vi "Filter and Data Scaling backup (062609) temp.vi"(0 "Offset Data":string[](array[string]), 1 "FM1 Frequency":dbl format="%#_13g", 5 "Slope Data":string[](array[string]), 7 "Filter Data":string[](array[string]), 9 "Vin":dbl[](array[numeric]), 11 "error in":errorcluster, 12 "Allow Zero?":string[](array[string])) -> (4 "Vout":string[](array[string]), 6 "Offset Data":string[](array[string]), 8 "ScaledOut":string[](array[string]), 10 "ScaledOut":dbl[](array[numeric]), 14 "Allow Zero?":string[](array[string]), 15 "error out":errorcluster)   [LabVIEW 2018]
uses:
  <vilib>/ptbypt/NI_PtbyPt.lvlib
panel:
  # "32-51= FM1 GPM Data Point 1-20"
  # "32-51= FM1 Data Point # 1-20"
  # "32-51 = FM1 K Factor 1-20"
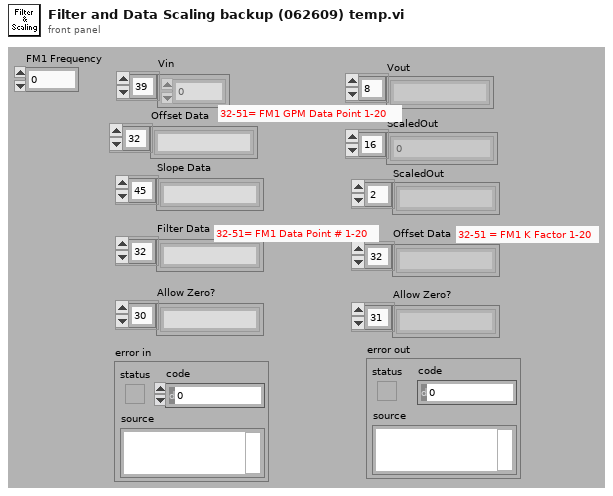
[diagram p1: front panel]
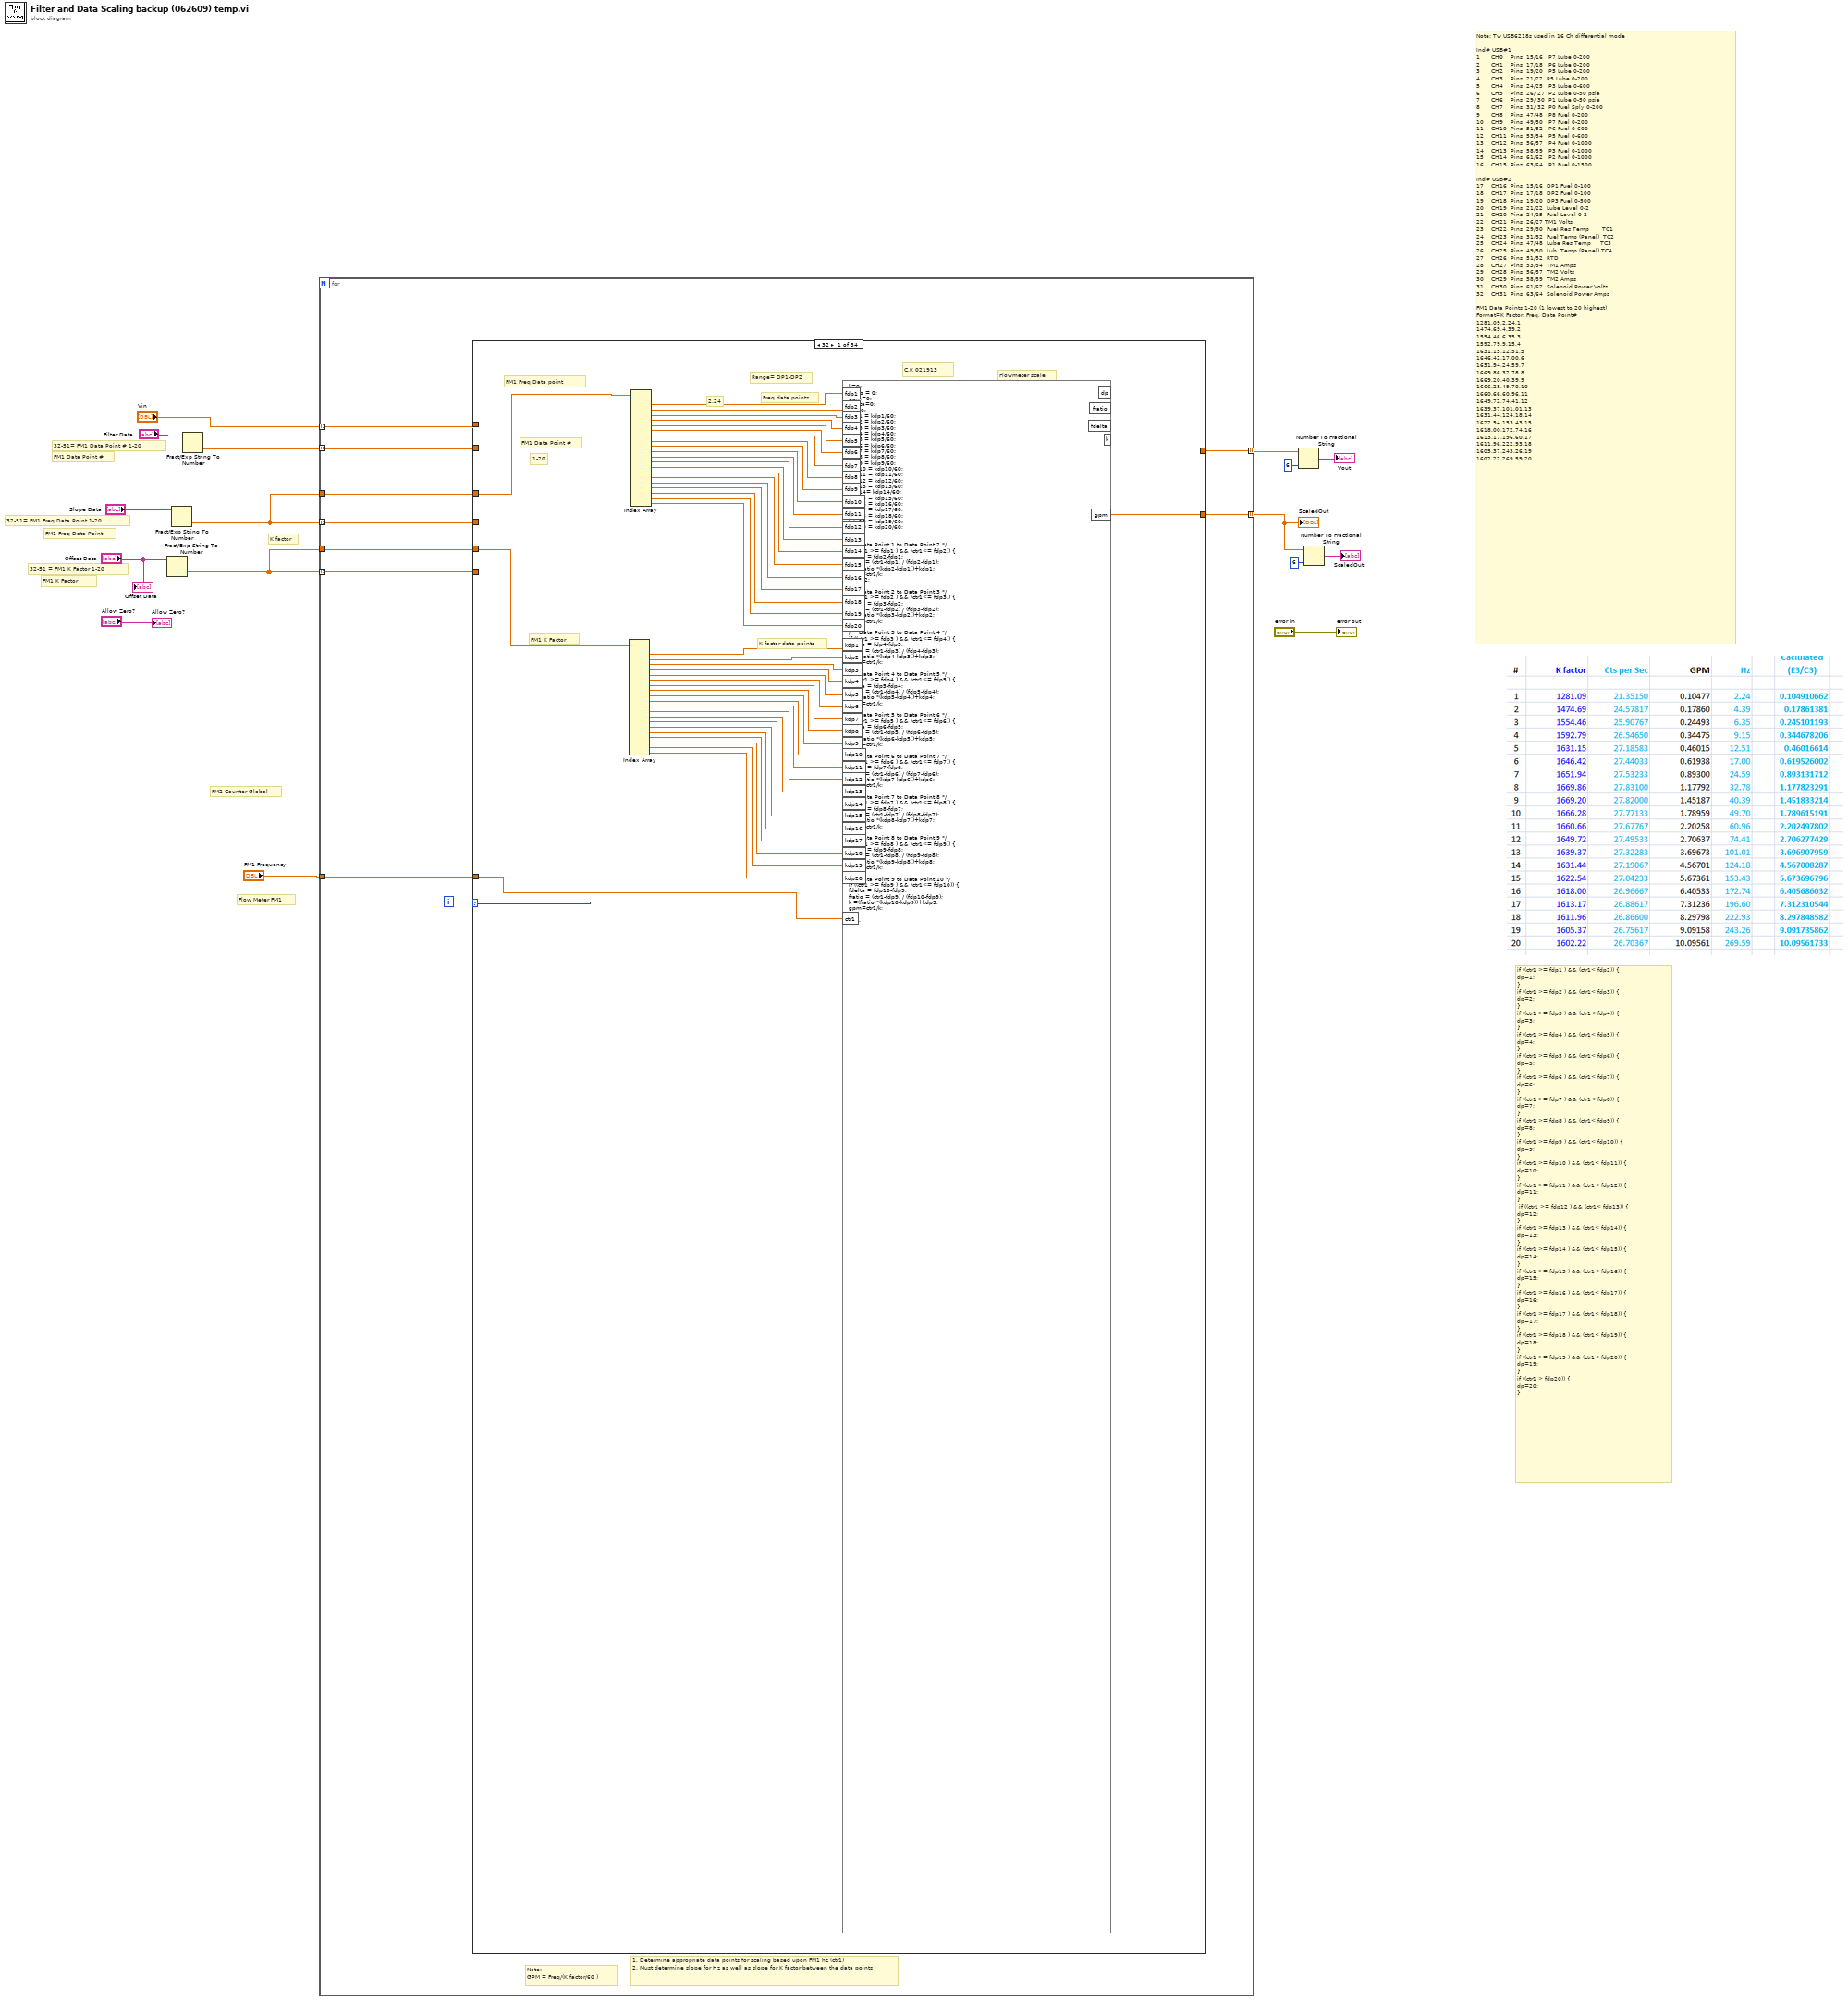
[diagram p0: block diagram]
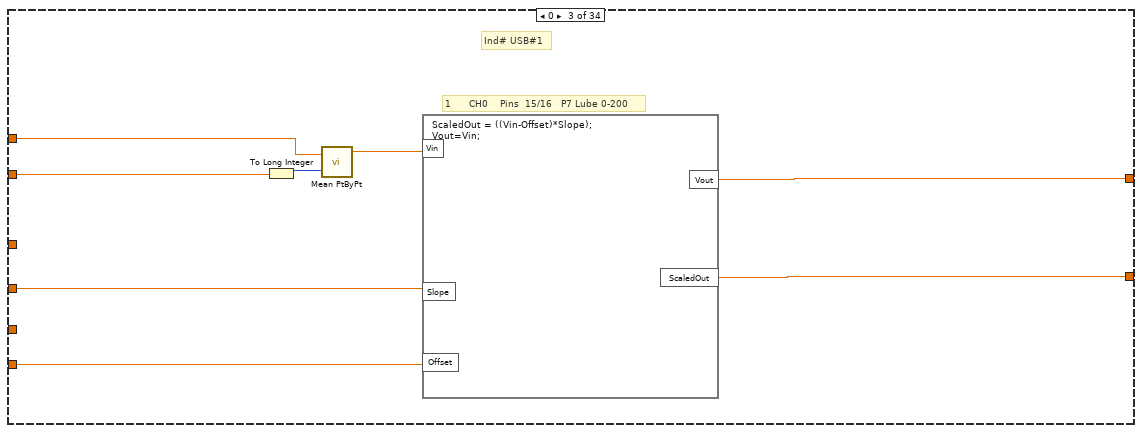
[diagram p3: hidden frame]
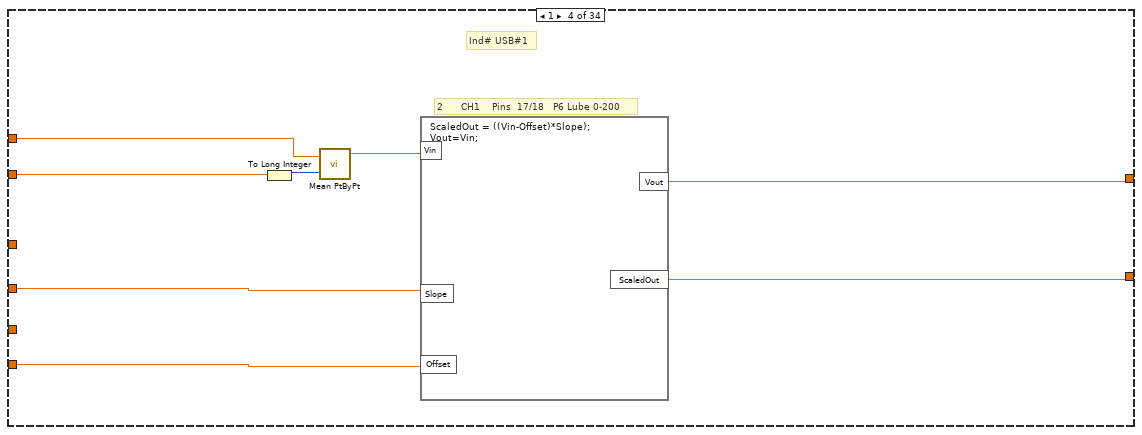
[diagram p4: hidden frame]
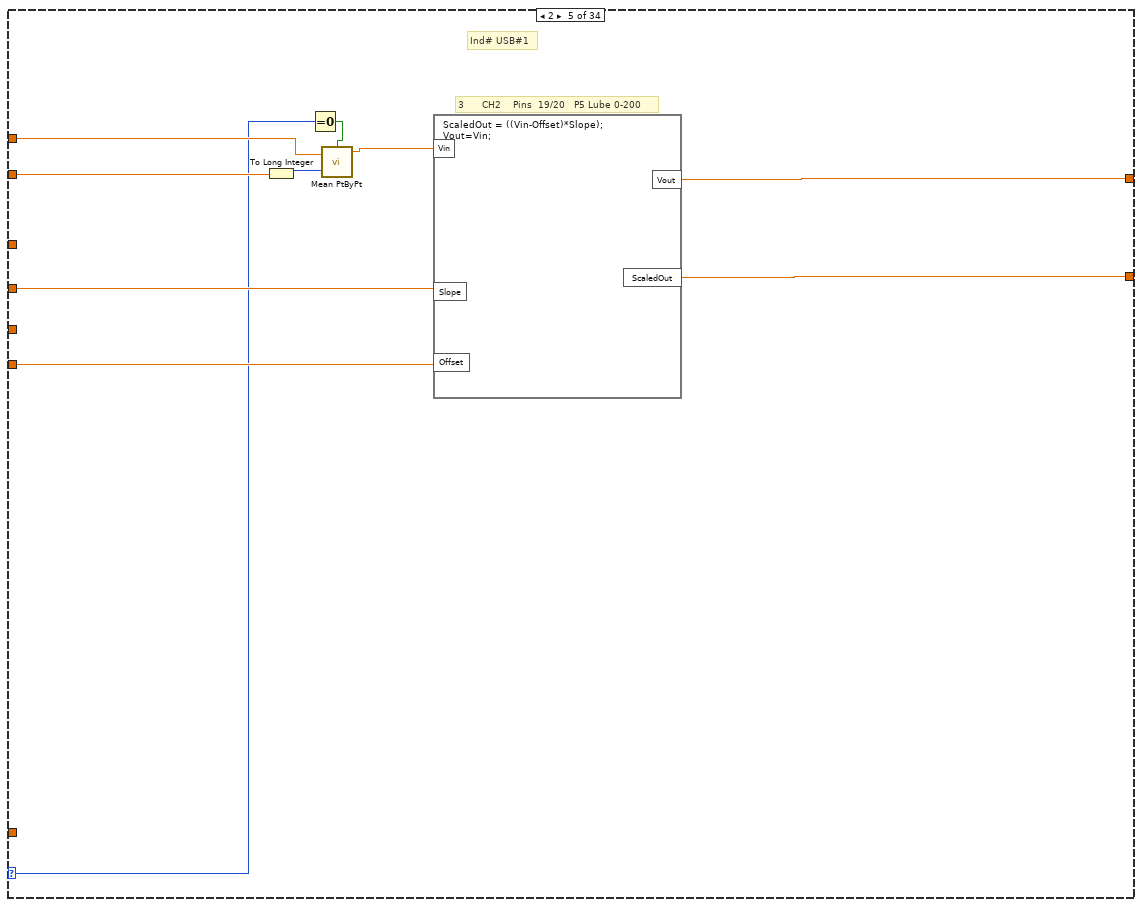
[diagram p5: hidden frame]
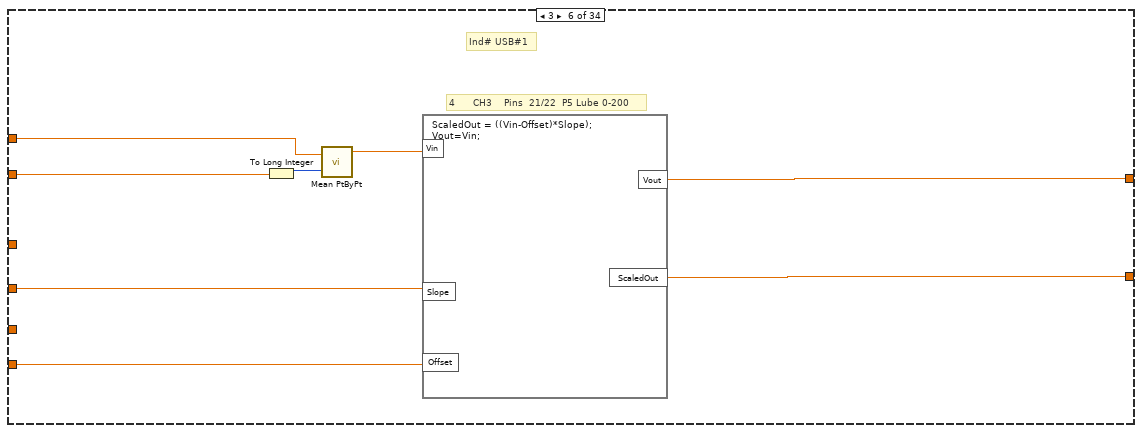
[diagram p6: hidden frame]
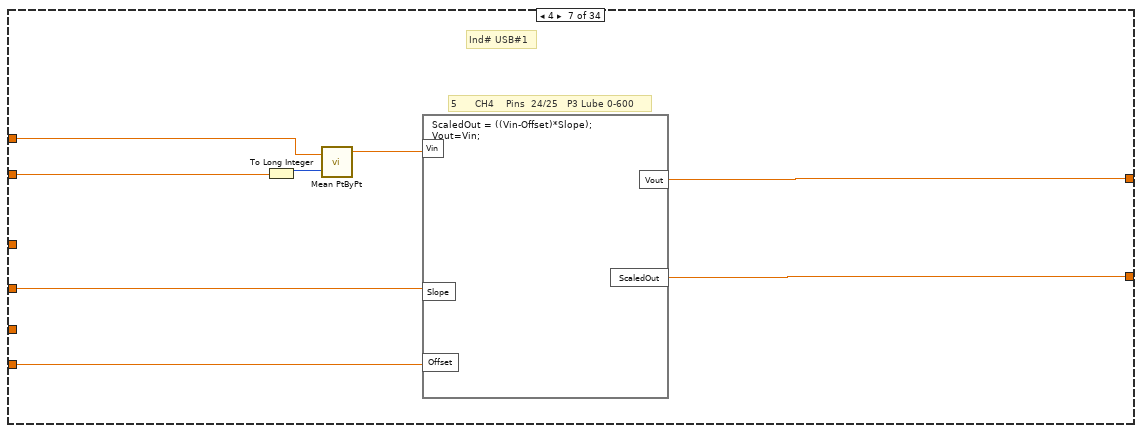
[diagram p7: hidden frame]
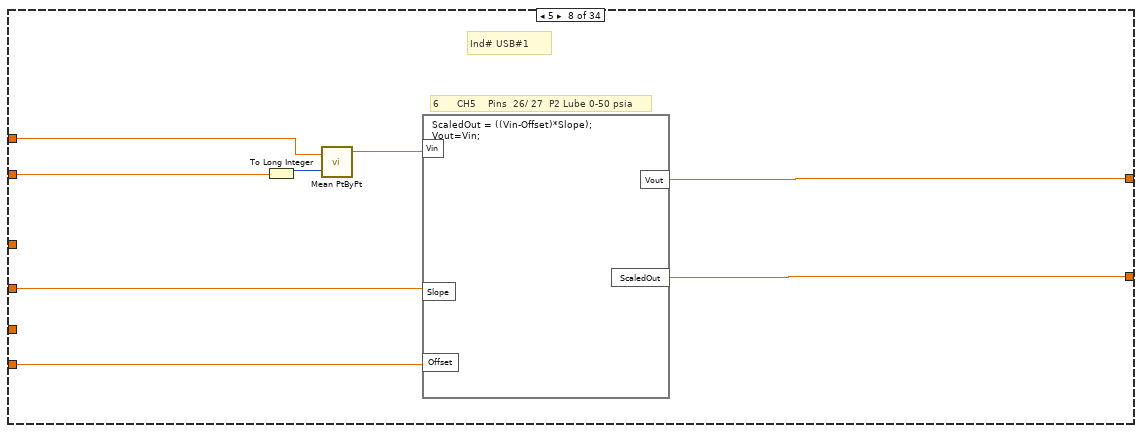
[diagram p8: hidden frame]
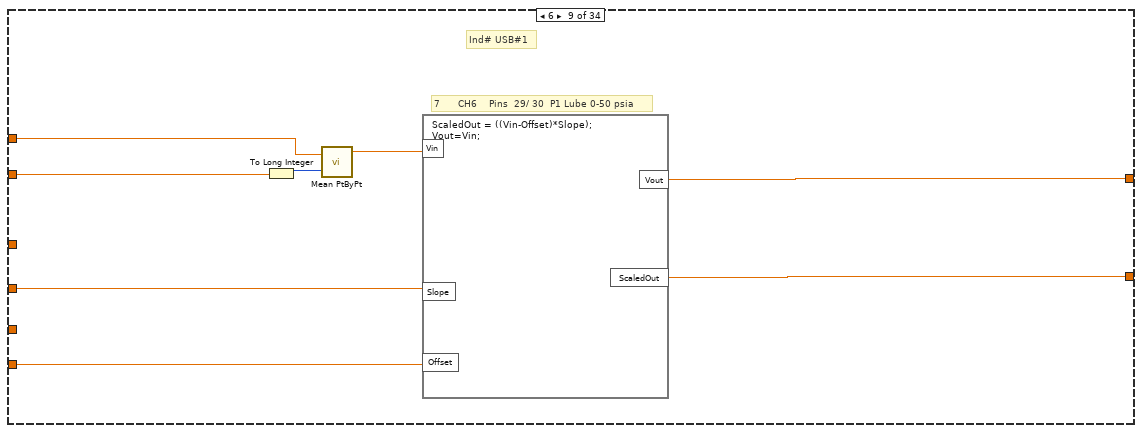
[diagram p9: hidden frame]
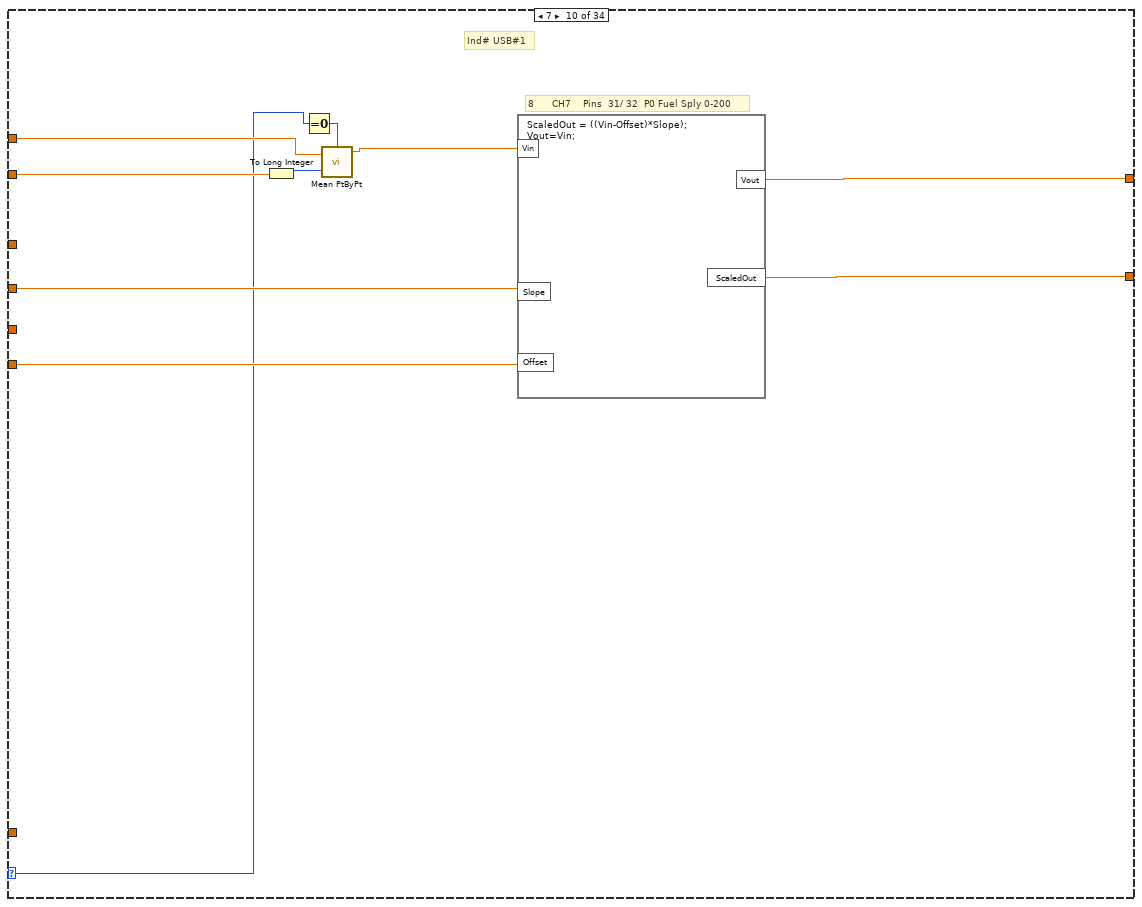
[diagram p10: hidden frame]
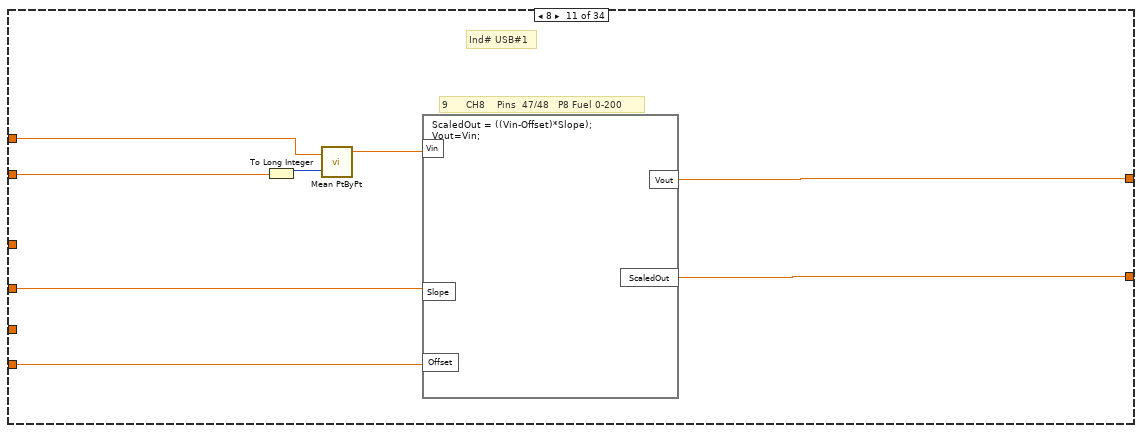
[diagram p11: hidden frame]
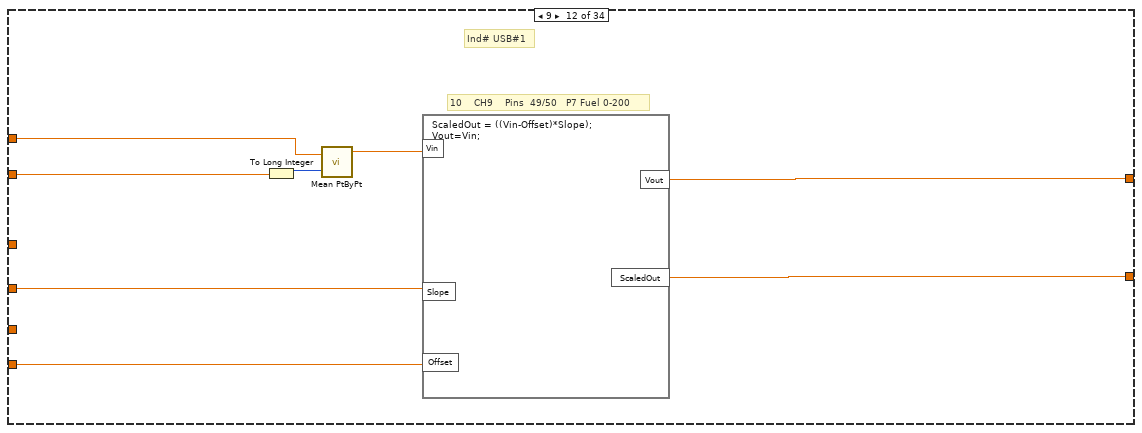
[diagram p12: hidden frame]
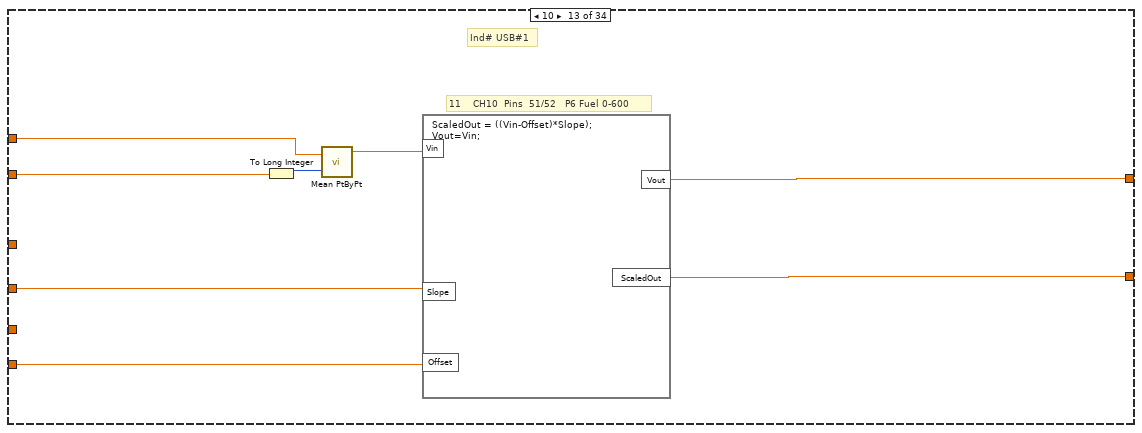
[diagram p13: hidden frame]
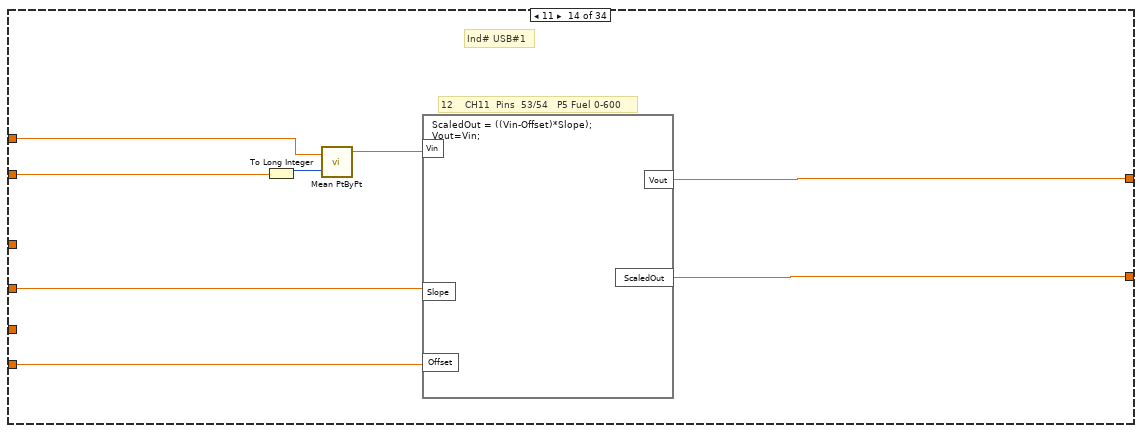
[diagram p14: hidden frame]
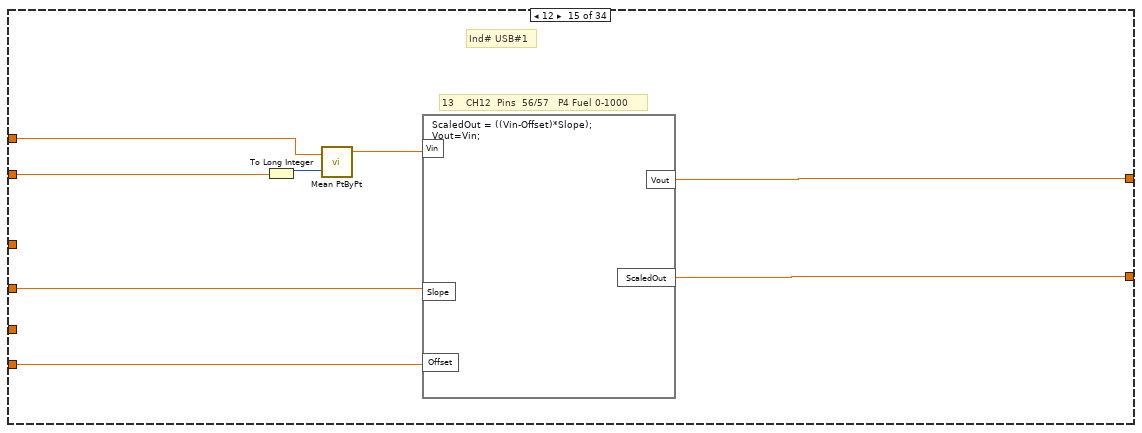
[diagram p15: hidden frame]
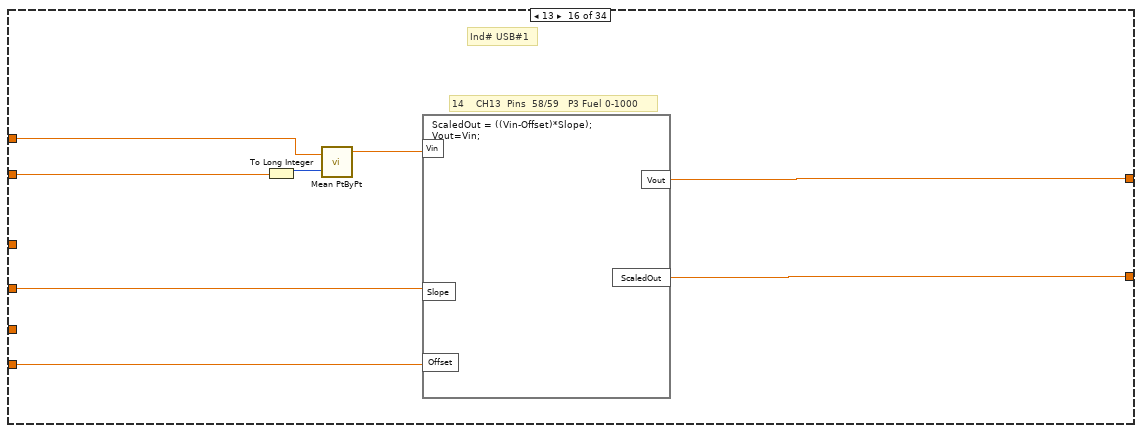
[diagram p16: hidden frame]
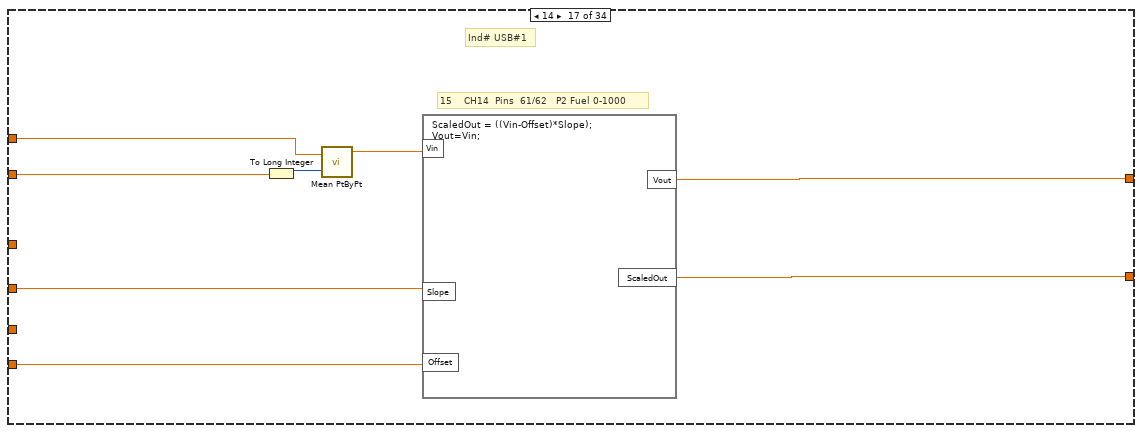
[diagram p17: hidden frame]
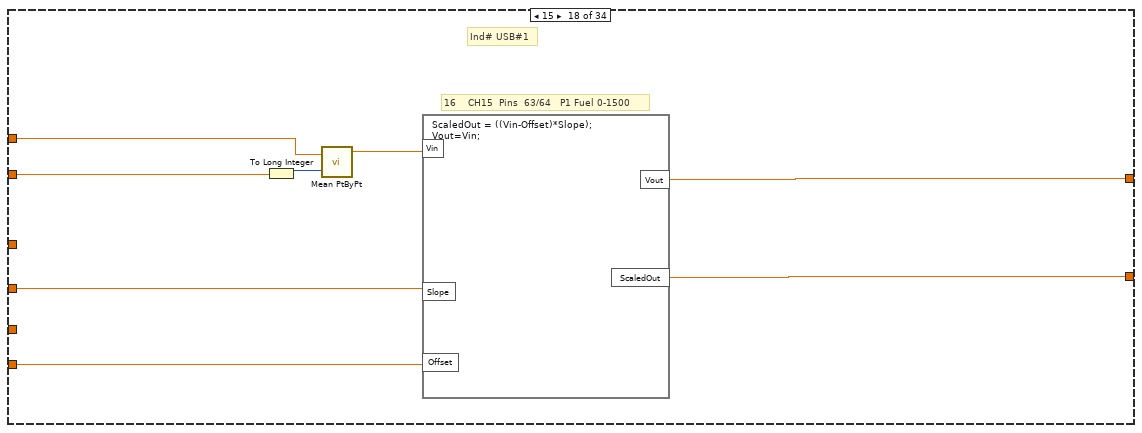
[diagram p18: hidden frame]
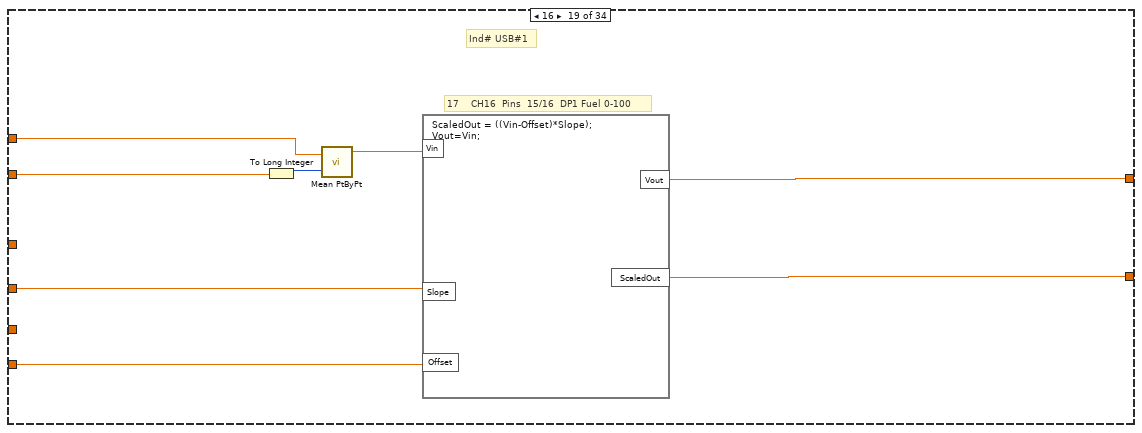
[diagram p19: hidden frame]
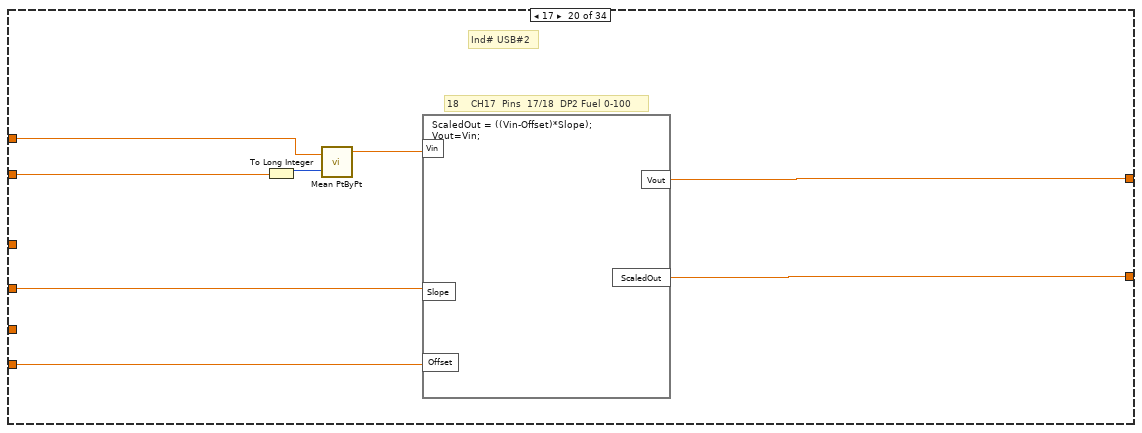
[diagram p20: hidden frame]
diagram:
  # "Flow Meter FM1"
  # "if ((ctr1 >= fdp1 ) && (ctr1< fdp2)) {\ndp=1;\n}\nif ((ctr1 >= fdp2 ) && (ctr1< fdp3)) {\ndp=2;\n}\nif ((ctr1 >= fdp3 ) && (ctr1< fdp4)) {\ndp=3;\n}\nif ((ctr1 >= fdp4 ) && (ctr1< fdp5)) {\ndp=4;\n}\nif ((ctr1 >= fdp5 ) && (ctr1< fdp6)) {\ndp=5;\n}\nif ((ctr1 >= fdp6 ) && (ctr1< fdp7)) {\ndp=6;\n}\nif ((ctr1 >= fdp7 ) && (ctr1< fdp8)) {\ndp=7;\n}\nif ((ctr1 >= fdp8 ) && (ctr1< fdp9)) {\ndp=8;\n}\nif ((ctr1 >= fdp9 ) && (ctr1< fdp10)) {\ndp=9;\n}\nif ((ctr1 >= fdp10 ) && (ctr1< fdp11)) {\ndp=10;\n}\nif ((ctr1 >= fdp11 ) && (ctr1< fdp12)) {\ndp=11;\n}\n if ((ctr1 >= fdp12 ) && (ctr1< fdp13)) {\ndp=12;\n}\nif ((ctr1 >= fdp13 ) && (ctr1< fdp14)) {\ndp=13;\n}\nif ((ctr1 >= fdp14 ) && (ctr1< fdp15)) {\ndp=14;\n}\nif ((ctr1 >= fdp15 ) && (ctr1< fdp16)) {\ndp=15;\n}\nif ((ctr1 >= fdp16 ) && (ctr1< fdp17)) {\ndp=16;\n}\nif ((ctr1 >= fdp17 ) && (ctr1< fdp18)) {\ndp=17;\n}\nif ((ctr1 >= fdp18 ) && (ctr1< fdp19)) {\ndp=18;\n}\nif ((ctr1 >= fdp19 ) && (ctr1< fdp20)) {\ndp=19;\n}\nif ((ctr1 > fdp20)) {\ndp=20;\n}"
  # "Note: Tw USB6218s used in 16 Ch differential mode\n\nInd# USB#1\n1      CH0\t\t  Pins  15/16\t  P7 Lube 0-200\n2      CH1\t\t  Pins  17/18\t  P6 Lube 0-200\n3      CH2\t\t  Pins  19/20   P5 Lube 0-200\n4      CH3\t\t  Pins  21/22  P5 Lube 0-200\n5      CH4\t   Pins  24/25\t  P3 Lube 0-600\n6      CH5\t\t  Pins  26/\t27\t P2 Lube 0-50 psia\n7      CH6\t   Pins  29/\t30\t P1 Lube 0-50 psia\n8      CH7\t  \tPins  31/ 32\t P0 Fuel Sply 0-200  \n9      CH8\t  \tPins  47/48\t  P8 Fuel 0-200   \n10    CH9\t\t  Pins  49/50\t  P7 Fuel 0-200   \n11    CH10\t\tPins  51/52\t  P6 Fuel 0-600   \n12    CH11\t\tPins  53/54\t  P5 Fuel 0-600   \n13    CH12\t\tPins  56/57\t  P4 Fuel 0-1000 \n14    CH13\t\tPins  58/59\t  P3 Fuel 0-1000 \n15    CH14\t\tPins  61/62 \t P2 Fuel 0-1000  \n16    CH15\t\tPins  63/64 \t P1 Fuel 0-1500 \n\nInd# USB#2\n17    CH16\t\tPins  15/16\t DP1 Fuel 0-100 \n18    CH17\t\tPins  17/18\t DP2 Fuel 0-100\n19    CH18\t\tPins  19/20  DP3 Fuel 0-500 \n20    CH19\t Pins  21/22\t Lube Level 0-2 \n21    CH20\t\tPins  24/25\t Fuel Level 0-2 \n22    CH21\t\tPins  26/27\tTM1 Volts  \n23    CH22\t Pins  29/30  Fuel Res Temp       TC1\n24    CH23\t\tPins  31/32\t Fuel Temp (Panel)  TC2 \n25    CH24\t\tPins \t47/48\t Lube Res Temp     TC3 \n26    CH25\t\tPins  49/50\t Lub  Temp (Panel) TC4 \n27    CH26\t\tPins  51/52\t RTD \n28    CH27\t\tPins  53/54\t TM1 Amps \n29    CH28\t\tPins  56/57\t TM2 Volts\n30    CH29\t\tPins  58/59\t TM2 Amps \n31    CH30\t\tPins  61/62  Solenoid Power Volts \n32    CH31\t\tPins  63/64  Solenoid Power Amps\n\nFM1 Data Points 1-20 (1 lowest to 20 highest)\nFormat=K Factor, Freq, Data Point#\n1281.09,2.24,1\n1474.69,4.39,2\n1554.46,6.35,3\n1592.79,9.15,4\n1631.15,12.51,5\n1646.42,17.00,6\n1651.94,24.59,7\n1669.86,32.78,8\n1669.20,40.39,9\n1666.28,49.70,10\n1660.66,60.96,11\n1649.72,74.41,12\n1639.37,101.01,13\n1631.44,124.18,14\n1622.54,153.43,15\n1618.00,172.74,16\n1613.17,196.60,17\n1611.96,222.93,18\n1605.37,243.26,19\n1602.22,269.59,20"
  # "K factor"
  # "FM1 Freq Data Point"
  # "FM2 Counter Global"
  # "FM1 Data Point #"
  # "FM1 K Factor"
  # "32-51 = FM1 K Factor 1-20"
  # "32-51= FM1 Data Point # 1-20"
  # "32-51= FM1 Freq Data Point 1-20"
  n1 = Fract/Exp String To Number(string="Offset Data") -> (number=w3:dbl[])  [unwired: 4 out]
  n2 = Fract/Exp String To Number(string="Slope Data") -> (number=w4:dbl[])  [unwired: 4 out]
  n3 = Fract/Exp String To Number(string="Filter Data") -> (number=w2:dbl[])  [unwired: 4 out]
  n4 = for {
    tunnel: w4 -> [w25] mode=indexing
    tunnel: w3 -> [w20] mode=indexing
    tunnel: w2 -> [w26] mode=indexing
    tunnel: [w23] -> w6 mode=indexing
    tunnel: [w24] -> w7 mode=indexing
    tunnel: "Vin" -> [w21] mode=indexing
    tunnel: w4 -> [w19]
    tunnel: w3 -> [w18]
    tunnel: "FM1 Frequency" -> [w17]
    i -> [w22]
    # "Note:\nGPM = Freq/(K factor/60 )"
    # "1. Determine appropriate data points for scaling based upon FM1 hz (ctr1)\n2. Must determine slope for Hz as well as slope for K factor between the data points"
    n5 = case shown="32" w22 {
      selector: w22 -> [_ _ _ _ w90 _ _ _ _ w132 _ _ _ _ _ _ _ _ _ _ _ _ _ _ _ _ _ _ _ _ _ _ _ _]
      tunnel: w21 -> [_ _ w75 w81 w95 w101 w109 w117 w125 w137 w143 w151 w159 w167 w175 w183 w191 w199 w207 w215 w223 w231 w239 w247 w255 w263 w271 w279 w287 w295 w303 w311 w319 w327]
      tunnel: w26 -> [_ _ w76 w82 w96 w102 w110 w118 w126 w138 w144 w152 w160 w168 w176 w184 w192 w200 w208 w216 w224 w232 w240 w248 w256 w264 w272 w280 w288 w296 w304 w312 w320 w328]
      tunnel: w25 -> [_ _ w74 w84 w94 w100 w108 w116 w124 w136 w142 w150 w158 w166 w174 w182 w190 w198 w206 w214 w222 w230 w238 w246 w254 w262 w270 w278 w286 w294 w302 w310 w318 w326]
      tunnel: w20 -> [_ _ w73 w83 w93 w99 w107 w115 w123 w135 w141 w149 w157 w165 w173 w181 w189 w197 w205 w213 w221 w229 w237 w245 w253 w261 w269 w277 w285 w293 w301 w309 w317 w325]
      tunnel: [_ _ w71 w80 w91 w97 w105 w113 w121 w133 w139 w147 w155 w163 w171 w179 w187 w195 w203 w211 w219 w227 w235 w244 w251 w259 w267 w275 w283 w292 w300 w308 w316 w324] -> w24
      tunnel: [w27 _ w72 w79 w92 w98 w106 w114 w122 w134 w140 w148 w156 w164 w172 w180 w188 w196 w204 w212 w220 w228 w236 w243 w252 w260 w268 w276 w284 w291 w299 w307 w315 w323] -> w23
      tunnel: w19 -> [w69 _ _ _ _ _ _ _ _ _ _ _ _ _ _ _ _ _ _ _ _ _ _ _ _ _ _ _ _ _ _ _ _ _]
      tunnel: w18 -> [w68 _ _ _ _ _ _ _ _ _ _ _ _ _ _ _ _ _ _ _ _ _ _ _ _ _ _ _ _ _ _ _ _ _]
      tunnel: w17 -> [w70 _ _ _ _ _ _ _ _ _ _ _ _ _ _ _ _ _ _ _ _ _ _ _ _ _ _ _ _ _ _ _ _ _]
      frame 32 {
        # "C.K 021913"
        # "2.24"
        # "Range= DP1-DP2"
        # "K factor data points"
        # "Freq data points"
        # "Flowmeter scale"
        # "1-20"
        # "FM1 Data Point #"
        # "FM1 K Factor"
        # "FM1 Freq Data point"
        n6 = Index Array(array=w68) -> (element #1=w47:dbl, element #2=w46:dbl, element #3=w45:dbl, element #4=w44:dbl, element #5=w43:dbl, element #6=w42:dbl, element #7=w41:dbl, element #8=w40:dbl, element #9=w39:dbl, element #10=w38:dbl, element #11=w37:dbl, element #12=w36:dbl, element #13=w35:dbl, element #14=w34:dbl, element #15=w33:dbl, element #16=w32:dbl, element #17=w31:dbl, element #18=w30:dbl, element #19=w29:dbl, element #20=w28:dbl)  [unwired: 20 in]
        n7 = Index Array(array=w69) -> (element #1=w67:dbl, element #2=w66:dbl, element #3=w65:dbl, element #4=w64:dbl, element #5=w63:dbl, element #6=w62:dbl, element #7=w61:dbl, element #8=w60:dbl, element #9=w59:dbl, element #10=w58:dbl, element #11=w57:dbl, element #12=w56:dbl, element #13=w55:dbl, element #14=w54:dbl, element #15=w53:dbl, element #16=w52:dbl, element #17=w51:dbl, element #18=w50:dbl, element #19=w49:dbl, element #20=w48:dbl)  [unwired: 20 in]
        n8 = formula code="k=0;\nfratio = 0;\ngpm=0;\nfdelta=0;\ndp=0;\nkdp1 = kdp1/60;\nkdp2 = kdp2/60;\nkdp3 = kdp3/60;\nkdp4 = kdp4/60;\nkdp5 = kdp5/60;\nkdp6 = kdp6/60;\nkdp7 = kdp7/60;\nkdp8 = kdp8/60;\nkdp9 = kdp9/60;\nkdp10 = kdp10/60;\nkdp11 = kdp11/60;\nkdp12 = kdp12/60;\nkdp13 = kdp13/60;\nkdp14= kdp14/60;\nkdp15 = kdp15/60;\nkdp16 = kdp16/60;\nkdp17 = kdp17/60;\nkdp18 = kdp18/60;\nkdp19 = kdp19/60;\nkdp20 = kdp20/60;\n\n\n/*   Data Point 1 to Data Point 2 */\nif ((ctr1 >= fdp1 ) && (ctr1<= fdp2)) {\nfdelta = fdp2-fdp1;\nfratio = (ctr1-fdp1) / (fdp2-fdp1);\nk =(fratio *(kdp2-kdp1))+kdp1;\ngpm=ctr1/k;\ndp=12;\n}\n/*   Data Point 2 to Data Point 3 */\nif ((ctr1 >= fdp2 ) && (ctr1<= fdp3)) {\nfdelta = fdp3-fdp2;\nfratio = (ctr1-fdp2) / (fdp3-fdp2);\nk =(fratio *(kdp3-kdp2))+kdp2;\ngpm=ctr1/k;\n}\n/*   Data Point 3 to Data Point 4 */\nif ((ctr1 >= fdp3 ) && (ctr1<= fdp4)) {\nfdelta = fdp4-fdp3;\nfratio = (ctr1-fdp3) / (fdp4-fdp3);\nk =(fratio *(kdp4-kdp3))+kdp3;\ngpm=ctr1/k;\n}\n/*   Data Point 4 to Data Point 5 */\nif ((ctr1 >= fdp4 ) && (ctr1<= fdp5)) {\nfdelta = fdp5-fdp4;\nfratio = (ctr1-fdp4) / (fdp5-fdp4);\nk =(fratio *(kdp5-kdp4))+kdp4;\ngpm=ctr1/k;\n}\n/*   Data Point 5 to Data Point 6 */\nif ((ctr1 >= fdp5 ) && (ctr1<= fdp6)) {\nfdelta = fdp6-fdp5;\nfratio = (ctr1-fdp5) / (fdp6-fdp5);\nk =(fratio *(kdp6-kdp5))+kdp5;\ngpm=ctr1/k;\n}\n/*   Data Point 6 to Data Point 7 */\nif ((ctr1 >= fdp6 ) && (ctr1<= fdp7)) {\nfdelta = fdp7-fdp6;\nfratio = (ctr1-fdp6) / (fdp7-fdp6);\nk =(fratio *(kdp7-kdp6))+kdp6;\ngpm=ctr1/k;\n}\n/*   Data Point 7 to Data Point 8 */\nif ((ctr1 >= fdp7 ) && (ctr1<= fdp8)) {\nfdelta = fdp8-fdp7;\nfratio = (ctr1-fdp7) / (fdp8-fdp7);\nk =(fratio *(kdp8-kdp7))+kdp7;\ngpm=ctr1/k;\n}\n/*   Data Point 8 to Data Point 9 */\nif ((ctr1 >= fdp8 ) && (ctr1<= fdp9)) {\nfdelta = fdp9-fdp8;\nfratio = (ctr1-fdp8) / (fdp9-fdp8);\nk =(fratio *(kdp9-kdp8))+kdp8;\ngpm=ctr1/k;\n}\n/*   Data Point 9 to Data Point 10 */\nif ((ctr1 >= fdp9 ) && (ctr1<= fdp10)) {\nfdelta = fdp10-fdp9;\nfratio = (ctr1-fdp9) / (fdp10-fdp9);\nk =(fratio *(kdp10-kdp9))+kdp9;\ngpm=ctr1/k;\n}\n/*   Data Point 10 to Data Point 11 */\nif ((ctr1 >= fdp10 ) && (ctr1<= fdp11)) {\nfdelta = fdp11-fdp10;\nfratio = (ctr1-fdp10) / (fdp11-fdp10);\nk =(fratio *(kdp11-kdp10))+kdp10;\ngpm=ctr1/k;\n}\n/*   Data Point 11 to Data Point 12 */\nif ((ctr1 >= fdp11 ) && (ctr1<= fdp12)) {\nfdelta = fdp12-fdp11;\nfratio = (ctr1-fdp11) / (fdp12-fdp11);\nk =(fratio *(kdp12-kdp11))+kdp11;\ngpm=ctr1/k;\n}\n/*   Data Point 12 to Data Point 13 */\nif ((ctr1 >= fdp12) && (ctr1<= fdp13)) {\nfdelta = fdp13-fdp12;\nfratio = (ctr1-fdp12) / (fdp13-fdp12);\nk =(fratio *(kdp13-kdp12))+kdp12;\ngpm=ctr1/k;\n}\n/*   Data Point 13 to Data Point 14 */\nif ((ctr1 >= fdp13 ) && (ctr1<= fdp14)) {\nfdelta = fdp14-fdp13;\nfratio = (ctr1-fdp13) / (fdp14-fdp13);\nk =(fratio *(kdp14-kdp13))+kdp13;\ngpm=ctr1/k;\n}\nif ((ctr1 >= fdp14 ) && (ctr1<= fdp15)) {\nfdelta = fdp15-fdp14;\nfratio = (ctr1-fdp14) / (fdp15-fdp14);\nk =(fratio *(kdp15-kdp14))+kdp14;\ngpm=ctr1/k;\n}\n/*   Data Point 15 to Data Point 16 */\nif ((ctr1 >= fdp15 ) && (ctr1<= fdp16)) {\nfdelta = fdp16-fdp15;\nfratio = (ctr1-fdp15) / (fdp16-fdp15);\nk =(fratio *(kdp16-kdp15))+kdp15;\ngpm=ctr1/k;\n}\n/*   Data Point 16 to Data Point 17 */\nif ((ctr1 >= fdp16 ) && (ctr1<= fdp17)) {\nfdelta = fdp17-fdp16;\nfratio = (ctr1-fdp16) / (fdp17-fdp16);\nk =(fratio *(kdp17-kdp16))+kdp16;\ngpm=ctr1/k;\n}\n/*   Data Point 17 to Data Point 18 */\nif ((ctr1 >= fdp17 ) && (ctr1<= fdp18)) {\nfdelta = fdp18-fdp17;\nfratio = (ctr1-fdp17) / (fdp18-fdp17);\nk =(fratio *(kdp18-kdp17))+kdp17;\ngpm=ctr1/k;\n}\n/*   Data Point 18 to Data Point 19 */\nif ((ctr1 >= fdp18 ) && (ctr1<= fdp19)) {\nfdelta = fdp19-fdp18;\nfratio = (ctr1-fdp18) / (fdp19-fdp18);\nk =(fratio *(kdp19-kdp18))+kdp18;\ngpm=ctr1/k;\n}\n/*   Data Point 19 to Data Point 20 */\nif ((ctr1 >= fdp19 ) && (ctr1<= fdp20)) {\nfdelta = fdp20-fdp19;\nfratio = (ctr1-fdp19) / (fdp20-fdp19);\nk =(fratio *(kdp20-kdp19))+kdp19;\ngpm=ctr1/k;\n}\nif (ctr1 >= fdp20) {\nfdelta = fdp20-fdp19;\nfratio = (ctr1-fdp19) / (fdp20-fdp19);\nk =(fratio *(kdp20-kdp19))+kdp19;\ngpm=ctr1/k;\ndp=2021;\n}\n\n/*   Data Point 0 to Data Point 1 temporary */\nif (ctr1 <= fdp1 ) {\nfdelta = fdp2-fdp1;\nfratio = (ctr1-fdp1) / (fdp2-fdp1);\nk =(fratio *(kdp2-kdp1))+kdp1;\ngpm=ctr1/k;\ndp=12;\n}"("fdp1"=w67, "fdp2"=w66, "kdp1"=w47, "ctr1"=w70, "kdp2"=w46, "fdp3"=w65, "fdp4"=w64, "fdp5"=w63, "fdp6"=w62, "fdp7"=w61, "fdp8"=w60, "fdp9"=w59, "fdp10"=w58, "fdp11"=w57, "fdp12"=w56, "fdp13"=w55, "fdp14"=w54, "fdp15"=w53, "fdp16"=w52, "fdp17"=w51, "fdp18"=w50, "fdp19"=w49, "fdp20"=w48, "kdp3"=w45, "kdp4"=w44, "kdp5"=w43, "kdp6"=w42, "kdp7"=w41, "kdp8"=w40, "kdp9"=w39, "kdp10"=w38, "kdp11"=w37, "kdp12"=w36, "kdp13"=w35, "kdp14"=w34, "kdp15"=w33, "kdp16"=w32, "kdp17"=w31, "kdp18"=w30, "kdp19"=w29, "kdp20"=w28) -> ("gpm"=w27:dbl)  [unwired: 4 out]
      }
      frame Default {
      }
      frame 0 {
        # "Ind# USB#1"
        # "1      CH0\t\t  Pins  15/16\t  P7 Lube 0-200"
        n9 = To Long Integer(number=w76) -> (32bit integer=w78:i32)
        n10 = call <vilib>:"Mean PtByPt.vi"("x"=w75, "sample length"=w78) -> ("mean"=w77:dbl)  [unwired: 1 in, 2 out]
        n11 = formula code="ScaledOut = ((Vin-Offset)*Slope);\nVout=Vin;"("Vin"=w77, "Slope"=w74, "Offset"=w73) -> ("ScaledOut"=w72:dbl, "Vout"=w71:dbl)
      }
      frame 1 {
        # "Ind# USB#1"
        # "2      CH1\t\t  Pins  17/18\t  P6 Lube 0-200"
        n12 = To Long Integer(number=w82) -> (32bit integer=w86:i32)
        n13 = call <vilib>:"Mean PtByPt.vi"("x"=w81, "sample length"=w86) -> ("mean"=w85:dbl)  [unwired: 1 in, 2 out]
        n14 = formula code="ScaledOut = ((Vin-Offset)*Slope);\nVout=Vin;"("Vin"=w85, "Slope"=w84, "Offset"=w83) -> ("ScaledOut"=w79:dbl, "Vout"=w80:dbl)
      }
      frame 2 {
        # "Ind# USB#1"
        # "3      CH2\t\t  Pins  19/20   P5 Lube 0-200"
        n15 = To Long Integer(number=w96) -> (32bit integer=w89:i32)
        n16 = Equal To 0?(x=w90) -> (x = 0?=w88:bool)
        n17 = call <vilib>:"Mean PtByPt.vi"("x"=w95, "sample length"=w89, "initialize"=w88) -> ("mean"=w87:dbl)  [unwired: 2 out]
        n18 = formula code="ScaledOut = ((Vin-Offset)*Slope);\nVout=Vin;"("Vin"=w87, "Slope"=w94, "Offset"=w93) -> ("ScaledOut"=w92:dbl, "Vout"=w91:dbl)
      }
      frame 3 {
        # "Ind# USB#1"
        # "4      CH3\t\t  Pins  21/22  P5 Lube 0-200"
        n19 = To Long Integer(number=w102) -> (32bit integer=w104:i32)
        n20 = call <vilib>:"Mean PtByPt.vi"("x"=w101, "sample length"=w104) -> ("mean"=w103:dbl)  [unwired: 1 in, 2 out]
        n21 = formula code="ScaledOut = ((Vin-Offset)*Slope);\nVout=Vin;"("Vin"=w103, "Slope"=w100, "Offset"=w99) -> ("ScaledOut"=w98:dbl, "Vout"=w97:dbl)
      }
      frame 4 {
        # "Ind# USB#1"
        # "5      CH4\t   Pins  24/25\t  P3 Lube 0-600"
        n22 = To Long Integer(number=w110) -> (32bit integer=w112:i32)
        n23 = call <vilib>:"Mean PtByPt.vi"("x"=w109, "sample length"=w112) -> ("mean"=w111:dbl)  [unwired: 1 in, 2 out]
        n24 = formula code="ScaledOut = ((Vin-Offset)*Slope);\nVout=Vin;"("Vin"=w111, "Slope"=w108, "Offset"=w107) -> ("ScaledOut"=w106:dbl, "Vout"=w105:dbl)
      }
      frame 5 {
        # "6      CH5\t\t  Pins  26/\t27\t P2 Lube 0-50 psia"
        # "Ind# USB#1"
        n25 = To Long Integer(number=w118) -> (32bit integer=w120:i32)
        n26 = call <vilib>:"Mean PtByPt.vi"("x"=w117, "sample length"=w120) -> ("mean"=w119:dbl)  [unwired: 1 in, 2 out]
        n27 = formula code="ScaledOut = ((Vin-Offset)*Slope);\nVout=Vin;"("Vin"=w119, "Slope"=w116, "Offset"=w115) -> ("ScaledOut"=w114:dbl, "Vout"=w113:dbl)
      }
      frame 6 {
        # "7      CH6\t   Pins  29/\t30\t P1 Lube 0-50 psia"
        # "Ind# USB#1"
        n28 = To Long Integer(number=w126) -> (32bit integer=w128:i32)
        n29 = call <vilib>:"Mean PtByPt.vi"("x"=w125, "sample length"=w128) -> ("mean"=w127:dbl)  [unwired: 1 in, 2 out]
        n30 = formula code="ScaledOut = ((Vin-Offset)*Slope);\nVout=Vin;"("Vin"=w127, "Slope"=w124, "Offset"=w123) -> ("ScaledOut"=w122:dbl, "Vout"=w121:dbl)
      }
      frame 7 {
        # "8      CH7\t  \tPins  31/ 32\t P0 Fuel Sply 0-200"
        # "Ind# USB#1"
        n31 = To Long Integer(number=w138) -> (32bit integer=w130:i32)
        n32 = Equal To 0?(x=w132) -> (x = 0?=w131:bool)
        n33 = call <vilib>:"Mean PtByPt.vi"("x"=w137, "sample length"=w130, "initialize"=w131) -> ("mean"=w129:dbl)  [unwired: 2 out]
        n34 = formula code="ScaledOut = ((Vin-Offset)*Slope);\nVout=Vin;"("Vin"=w129, "Slope"=w136, "Offset"=w135) -> ("ScaledOut"=w134:dbl, "Vout"=w133:dbl)
      }
      frame 8 {
        # "9      CH8\t  \tPins  47/48\t  P8 Fuel 0-200"
        # "Ind# USB#1"
        n35 = To Long Integer(number=w144) -> (32bit integer=w146:i32)
        n36 = call <vilib>:"Mean PtByPt.vi"("x"=w143, "sample length"=w146) -> ("mean"=w145:dbl)  [unwired: 1 in, 2 out]
        n37 = formula code="ScaledOut = ((Vin-Offset)*Slope);\nVout=Vin;"("Vin"=w145, "Slope"=w142, "Offset"=w141) -> ("ScaledOut"=w140:dbl, "Vout"=w139:dbl)
      }
      frame 9 {
        # "10    CH9\t\t  Pins  49/50\t  P7 Fuel 0-200"
        # "Ind# USB#1"
        n38 = To Long Integer(number=w152) -> (32bit integer=w154:i32)
        n39 = call <vilib>:"Mean PtByPt.vi"("x"=w151, "sample length"=w154) -> ("mean"=w153:dbl)  [unwired: 1 in, 2 out]
        n40 = formula code="ScaledOut = ((Vin-Offset)*Slope);\nVout=Vin;"("Vin"=w153, "Slope"=w150, "Offset"=w149) -> ("ScaledOut"=w148:dbl, "Vout"=w147:dbl)
      }
      frame 10 {
        # "11    CH10\t\tPins  51/52\t  P6 Fuel 0-600"
        # "Ind# USB#1"
        n41 = To Long Integer(number=w160) -> (32bit integer=w162:i32)
        n42 = call <vilib>:"Mean PtByPt.vi"("x"=w159, "sample length"=w162) -> ("mean"=w161:dbl)  [unwired: 1 in, 2 out]
        n43 = formula code="ScaledOut = ((Vin-Offset)*Slope);\nVout=Vin;"("Vin"=w161, "Slope"=w158, "Offset"=w157) -> ("ScaledOut"=w156:dbl, "Vout"=w155:dbl)
      }
      frame 11 {
        # "12    CH11\t\tPins  53/54\t  P5 Fuel 0-600"
        # "Ind# USB#1"
        n44 = To Long Integer(number=w168) -> (32bit integer=w170:i32)
        n45 = call <vilib>:"Mean PtByPt.vi"("x"=w167, "sample length"=w170) -> ("mean"=w169:dbl)  [unwired: 1 in, 2 out]
        n46 = formula code="ScaledOut = ((Vin-Offset)*Slope);\nVout=Vin;"("Vin"=w169, "Slope"=w166, "Offset"=w165) -> ("ScaledOut"=w164:dbl, "Vout"=w163:dbl)
      }
      frame 12 {
        # "13    CH12\t\tPins  56/57\t  P4 Fuel 0-1000"
        # "Ind# USB#1"
        n47 = To Long Integer(number=w176) -> (32bit integer=w178:i32)
        n48 = call <vilib>:"Mean PtByPt.vi"("x"=w175, "sample length"=w178) -> ("mean"=w177:dbl)  [unwired: 1 in, 2 out]
        n49 = formula code="ScaledOut = ((Vin-Offset)*Slope);\nVout=Vin;"("Vin"=w177, "Slope"=w174, "Offset"=w173) -> ("ScaledOut"=w172:dbl, "Vout"=w171:dbl)
      }
      frame 13 {
        # "14    CH13\t\tPins  58/59\t  P3 Fuel 0-1000"
        # "Ind# USB#1"
        n50 = To Long Integer(number=w184) -> (32bit integer=w186:i32)
        n51 = call <vilib>:"Mean PtByPt.vi"("x"=w183, "sample length"=w186) -> ("mean"=w185:dbl)  [unwired: 1 in, 2 out]
        n52 = formula code="ScaledOut = ((Vin-Offset)*Slope);\nVout=Vin;"("Vin"=w185, "Slope"=w182, "Offset"=w181) -> ("ScaledOut"=w180:dbl, "Vout"=w179:dbl)
      }
      frame 14 {
        # "15    CH14\t\tPins  61/62 \t P2 Fuel 0-1000"
        # "Ind# USB#1"
        n53 = To Long Integer(number=w192) -> (32bit integer=w194:i32)
        n54 = call <vilib>:"Mean PtByPt.vi"("x"=w191, "sample length"=w194) -> ("mean"=w193:dbl)  [unwired: 1 in, 2 out]
        n55 = formula code="ScaledOut = ((Vin-Offset)*Slope);\nVout=Vin;"("Vin"=w193, "Slope"=w190, "Offset"=w189) -> ("ScaledOut"=w188:dbl, "Vout"=w187:dbl)
      }
      frame 15 {
        # "16    CH15\t\tPins  63/64 \t P1 Fuel 0-1500"
        # "Ind# USB#1"
        n56 = To Long Integer(number=w200) -> (32bit integer=w202:i32)
        n57 = call <vilib>:"Mean PtByPt.vi"("x"=w199, "sample length"=w202) -> ("mean"=w201:dbl)  [unwired: 1 in, 2 out]
        n58 = formula code="ScaledOut = ((Vin-Offset)*Slope);\nVout=Vin;"("Vin"=w201, "Slope"=w198, "Offset"=w197) -> ("ScaledOut"=w196:dbl, "Vout"=w195:dbl)
      }
      frame 16 {
        # "17    CH16\t\tPins  15/16\t DP1 Fuel 0-100"
        # "Ind# USB#1"
        n59 = To Long Integer(number=w208) -> (32bit integer=w210:i32)
        n60 = call <vilib>:"Mean PtByPt.vi"("x"=w207, "sample length"=w210) -> ("mean"=w209:dbl)  [unwired: 1 in, 2 out]
        n61 = formula code="ScaledOut = ((Vin-Offset)*Slope);\nVout=Vin;"("Vin"=w209, "Slope"=w206, "Offset"=w205) -> ("ScaledOut"=w204:dbl, "Vout"=w203:dbl)
      }
      frame 17 {
        # "18    CH17\t\tPins  17/18\t DP2 Fuel 0-100"
        # "Ind# USB#2"
        n62 = To Long Integer(number=w216) -> (32bit integer=w218:i32)
        n63 = call <vilib>:"Mean PtByPt.vi"("x"=w215, "sample length"=w218) -> ("mean"=w217:dbl)  [unwired: 1 in, 2 out]
        n64 = formula code="ScaledOut = ((Vin-Offset)*Slope);\nVout=Vin;"("Vin"=w217, "Slope"=w214, "Offset"=w213) -> ("ScaledOut"=w212:dbl, "Vout"=w211:dbl)
      }
      frame 18 {
        # "19    CH18\t\tPins  19/20  DP3 Fuel 0-500"
        # "Ind# USB#2"
        n65 = To Long Integer(number=w224) -> (32bit integer=w226:i32)
        n66 = call <vilib>:"Mean PtByPt.vi"("x"=w223, "sample length"=w226) -> ("mean"=w225:dbl)  [unwired: 1 in, 2 out]
        n67 = formula code="ScaledOut = ((Vin-Offset)*Slope);\nVout=Vin;"("Vin"=w225, "Slope"=w222, "Offset"=w221) -> ("ScaledOut"=w220:dbl, "Vout"=w219:dbl)
      }
      frame 19 {
        # "20    CH19\t Pins  21/22\t Lube Level 0-2"
        # "Ind# USB#2"
        n68 = To Long Integer(number=w232) -> (32bit integer=w234:i32)
        n69 = call <vilib>:"Mean PtByPt.vi"("x"=w231, "sample length"=w234) -> ("mean"=w233:dbl)  [unwired: 1 in, 2 out]
        n70 = formula code="ScaledOut = ((Vin-Offset)*Slope);\nVout=Vin;"("Vin"=w233, "Slope"=w230, "Offset"=w229) -> ("ScaledOut"=w228:dbl, "Vout"=w227:dbl)
      }
      frame 20 {
        # "21    CH20\t\tPins  24/25\t Fuel Level 0-2"
        # "Ind# USB#2"
        n71 = To Long Integer(number=w240) -> (32bit integer=w242:i32)
        n72 = call <vilib>:"Mean PtByPt.vi"("x"=w239, "sample length"=w242) -> ("mean"=w241:dbl)  [unwired: 1 in, 2 out]
        n73 = formula code="ScaledOut = ((Vin-Offset)*Slope);\nVout=Vin;"("Vin"=w241, "Slope"=w238, "Offset"=w237) -> ("ScaledOut"=w236:dbl, "Vout"=w235:dbl)
      }
      frame 21 {
        # "22    CH21\t\tPins  26/27\tTM1 Volts"
        # "Ind# USB#2"
        n74 = To Long Integer(number=w248) -> (32bit integer=w250:i32)
        n75 = call <vilib>:"Mean PtByPt.vi"("x"=w247, "sample length"=w250) -> ("mean"=w249:dbl)  [unwired: 1 in, 2 out]
        n76 = formula code="ScaledOut = ((Vin-Offset)*Slope);\nVout=Vin;"("Vin"=w249, "Slope"=w246, "Offset"=w245) -> ("ScaledOut"=w243:dbl, "Vout"=w244:dbl)
      }
      frame 22 {
        # "23    CH22\t Pins  29/30  Fuel Res Temp       TC1"
        # "Ind# USB#2"
        n77 = To Long Integer(number=w256) -> (32bit integer=w258:i32)
        n78 = call <vilib>:"Mean PtByPt.vi"("x"=w255, "sample length"=w258) -> ("mean"=w257:dbl)  [unwired: 1 in, 2 out]
        n79 = formula code="ScaledOut = ((Vin-Offset)*Slope);\nVout=Vin;"("Vin"=w257, "Slope"=w254, "Offset"=w253) -> ("ScaledOut"=w252:dbl, "Vout"=w251:dbl)
      }
      frame 23 {
        # "24    CH23\t\tPins  31/32\t Fuel Temp (Panel)  TC2"
        # "Ind# USB#2"
        n80 = To Long Integer(number=w264) -> (32bit integer=w266:i32)
        n81 = call <vilib>:"Mean PtByPt.vi"("x"=w263, "sample length"=w266) -> ("mean"=w265:dbl)  [unwired: 1 in, 2 out]
        n82 = formula code="ScaledOut = ((Vin-Offset)*Slope);\nVout=Vin;"("Vin"=w265, "Slope"=w262, "Offset"=w261) -> ("ScaledOut"=w260:dbl, "Vout"=w259:dbl)
      }
      frame 24 {
        # "25    CH24\t\tPins \t47/48\t Lube Res Temp     TC3"
        # "Ind# USB#2"
        n83 = To Long Integer(number=w272) -> (32bit integer=w274:i32)
        n84 = call <vilib>:"Mean PtByPt.vi"("x"=w271, "sample length"=w274) -> ("mean"=w273:dbl)  [unwired: 1 in, 2 out]
        n85 = formula code="ScaledOut = ((Vin-Offset)*Slope);\nVout=Vin;"("Vin"=w273, "Slope"=w270, "Offset"=w269) -> ("ScaledOut"=w268:dbl, "Vout"=w267:dbl)
      }
      frame 25 {
        # "26    CH25\t\tPins  49/50\t Lub  Temp (Panel) TC4"
        # "Ind# USB#2"
        n86 = To Long Integer(number=w280) -> (32bit integer=w282:i32)
        n87 = call <vilib>:"Mean PtByPt.vi"("x"=w279, "sample length"=w282) -> ("mean"=w281:dbl)  [unwired: 1 in, 2 out]
        n88 = formula code="ScaledOut = ((Vin-Offset)*Slope);\nVout=Vin;"("Vin"=w281, "Slope"=w278, "Offset"=w277) -> ("ScaledOut"=w276:dbl, "Vout"=w275:dbl)
      }
      frame 26 {
        # "27    CH26\t\tPins  51/52\t RTD"
        # "Ind# USB#2"
        n89 = To Long Integer(number=w288) -> (32bit integer=w290:i32)
        n90 = call <vilib>:"Mean PtByPt.vi"("x"=w287, "sample length"=w290) -> ("mean"=w289:dbl)  [unwired: 1 in, 2 out]
        n91 = formula code="ScaledOut = ((Vin-Offset)*Slope);\nVout=Vin;"("Vin"=w289, "Slope"=w286, "Offset"=w285) -> ("ScaledOut"=w284:dbl, "Vout"=w283:dbl)
      }
      frame 27 {
        # "28    CH27\t\tPins  53/54\t TM1 Amps"
        # "Ind# USB#2"
        n92 = To Long Integer(number=w296) -> (32bit integer=w298:i32)
        n93 = call <vilib>:"Mean PtByPt.vi"("x"=w295, "sample length"=w298) -> ("mean"=w297:dbl)  [unwired: 1 in, 2 out]
        n94 = formula code="ScaledOut = ((Vin-Offset)*Slope);\nVout=Vin;"("Vin"=w297, "Slope"=w294, "Offset"=w293) -> ("ScaledOut"=w291:dbl, "Vout"=w292:dbl)
      }
      frame 28 {
        # "29    CH28\t\tPins  56/57\t TM2 Volts"
        # "Ind# USB#2"
        n95 = To Long Integer(number=w304) -> (32bit integer=w306:i32)
        n96 = call <vilib>:"Mean PtByPt.vi"("x"=w303, "sample length"=w306) -> ("mean"=w305:dbl)  [unwired: 1 in, 2 out]
        n97 = formula code="ScaledOut = ((Vin-Offset)*Slope);\nVout=Vin;"("Vin"=w305, "Slope"=w302, "Offset"=w301) -> ("ScaledOut"=w299:dbl, "Vout"=w300:dbl)
      }
      frame 29 {
        # "30    CH29\t\tPins  58/59\t TM2 Amps"
        # "Ind# USB#2"
        n98 = To Long Integer(number=w312) -> (32bit integer=w314:i32)
        n99 = call <vilib>:"Mean PtByPt.vi"("x"=w311, "sample length"=w314) -> ("mean"=w313:dbl)  [unwired: 1 in, 2 out]
        n100 = formula code="ScaledOut = ((Vin-Offset)*Slope);\nVout=Vin;"("Vin"=w313, "Slope"=w310, "Offset"=w309) -> ("ScaledOut"=w307:dbl, "Vout"=w308:dbl)
      }
      frame 30 {
        # "31    CH30\t\tPins  61/62  Solenoid Power Volts"
        # "Ind# USB#2"
        n101 = To Long Integer(number=w320) -> (32bit integer=w322:i32)
        n102 = call <vilib>:"Mean PtByPt.vi"("x"=w319, "sample length"=w322) -> ("mean"=w321:dbl)  [unwired: 1 in, 2 out]
        n103 = formula code="ScaledOut = ((Vin-Offset)*Slope);\nVout=Vin;"("Vin"=w321, "Slope"=w318, "Offset"=w317) -> ("ScaledOut"=w315:dbl, "Vout"=w316:dbl)
      }
      frame 31 {
        # "32    CH31\t\tPins  63/64  Solenoid Power Amps"
        # "Ind# USB#2"
        n104 = To Long Integer(number=w328) -> (32bit integer=w330:i32)
        n105 = call <vilib>:"Mean PtByPt.vi"("x"=w327, "sample length"=w330) -> ("mean"=w329:dbl)  [unwired: 1 in, 2 out]
        n106 = formula code="ScaledOut = ((Vin-Offset)*Slope);\nVout=Vin;"("Vin"=w329, "Slope"=w326, "Offset"=w325) -> ("ScaledOut"=w323:dbl, "Vout"=w324:dbl)
      }
    }
  }
  "ScaledOut" <- w6
  n107 = Number To Fractional String(number=w7, precision (6)=i16 6) -> (F-format string=→"Vout":string[])  [unwired: 2 out]
  n108 = Number To Fractional String(number=w6, precision (6)=i16 6) -> (F-format string=→"ScaledOut":string[])  [unwired: 2 out]
  "Allow Zero?" <- "Allow Zero?"
  "Offset Data" <- "Offset Data"
  "error out" <- "error in"
